vi "only_ang.vi"(9 "wanted angle":dbl=-36.7) -> ()   [LabVIEW 2019]
uses:
  <vilib>/Platform/TimedLoop/XDataNode/timing_clust.ctl
  <vilib>/Platform/TimedLoop/XDataNode/nitl_modes.ctl
  <vilib>/Platform/TimedLoop/XDataNode/wakeup.ctl
  <vilib>/FPGAPlugInAG/myRIO-1900/niLvFpga_Open_myRIO-1900.vi
  <vilib>/rvi/interface/common/dynamic/niFpgaDynamicAddResources.vi
  <vilib>/Utility/error.llb/Error Cluster From Error Code.vi
  <vilib>/rvi/errors/niLvFpgaAdjustHostInterfaceError.vi
  <vilib>/FPGAPlugInAG/Dynamic/niLvFpga_Close_Dynamic.vi
  <vilib>/rvi/interface/nirviOpenFPGA/nirviOpenFPGA.xnode
  FPGA Bitfiles/capstone_FPGATarget_FPGA(test)_jvt0Tj5QNIc.lvbitx
  FPGA(test)_.vi
  <vilib>/rvi/interface/nirviReadWriteControl/nirviReadWriteControl.xnode
  <vilib>/Platform/TimedLoop/XDataNode/XDataNode.xnode
  <vilib>/rvi/interface/nirviCloseFPGA/nirviCloseFPGA.xnode
  <vilib>/Platform/TimedLoop/XDataNode/XDNodeRunTimeDep.lvlib
  <vilib>/rvi/interface/Simulation/niFpgaSimulationCallBeginRW.vi
  NiFpgaLv.dll
panel:
  out "reference":cluster{"wanted angle":dbl, dbl}(graph)={"wanted angle"=-36.7, -36.61462118459303}
  in  "Ki":dbl=50.0
  out "pwm_out":i32
  in  "Kd":dbl=0.01
  out "방향":bool
  in  "stop":bool
  in  "Enable (escon)":bool
  out "u(k) = pwm":dbl
  in  "Kp":dbl=500.0
  out "now angle":dbl
  out "Now mot rev":dbl
  out "Timeout":i32=-1
  out "Encoder  (4x)":i32
  # "쓰지마"
  # "----마이너스------해야함"
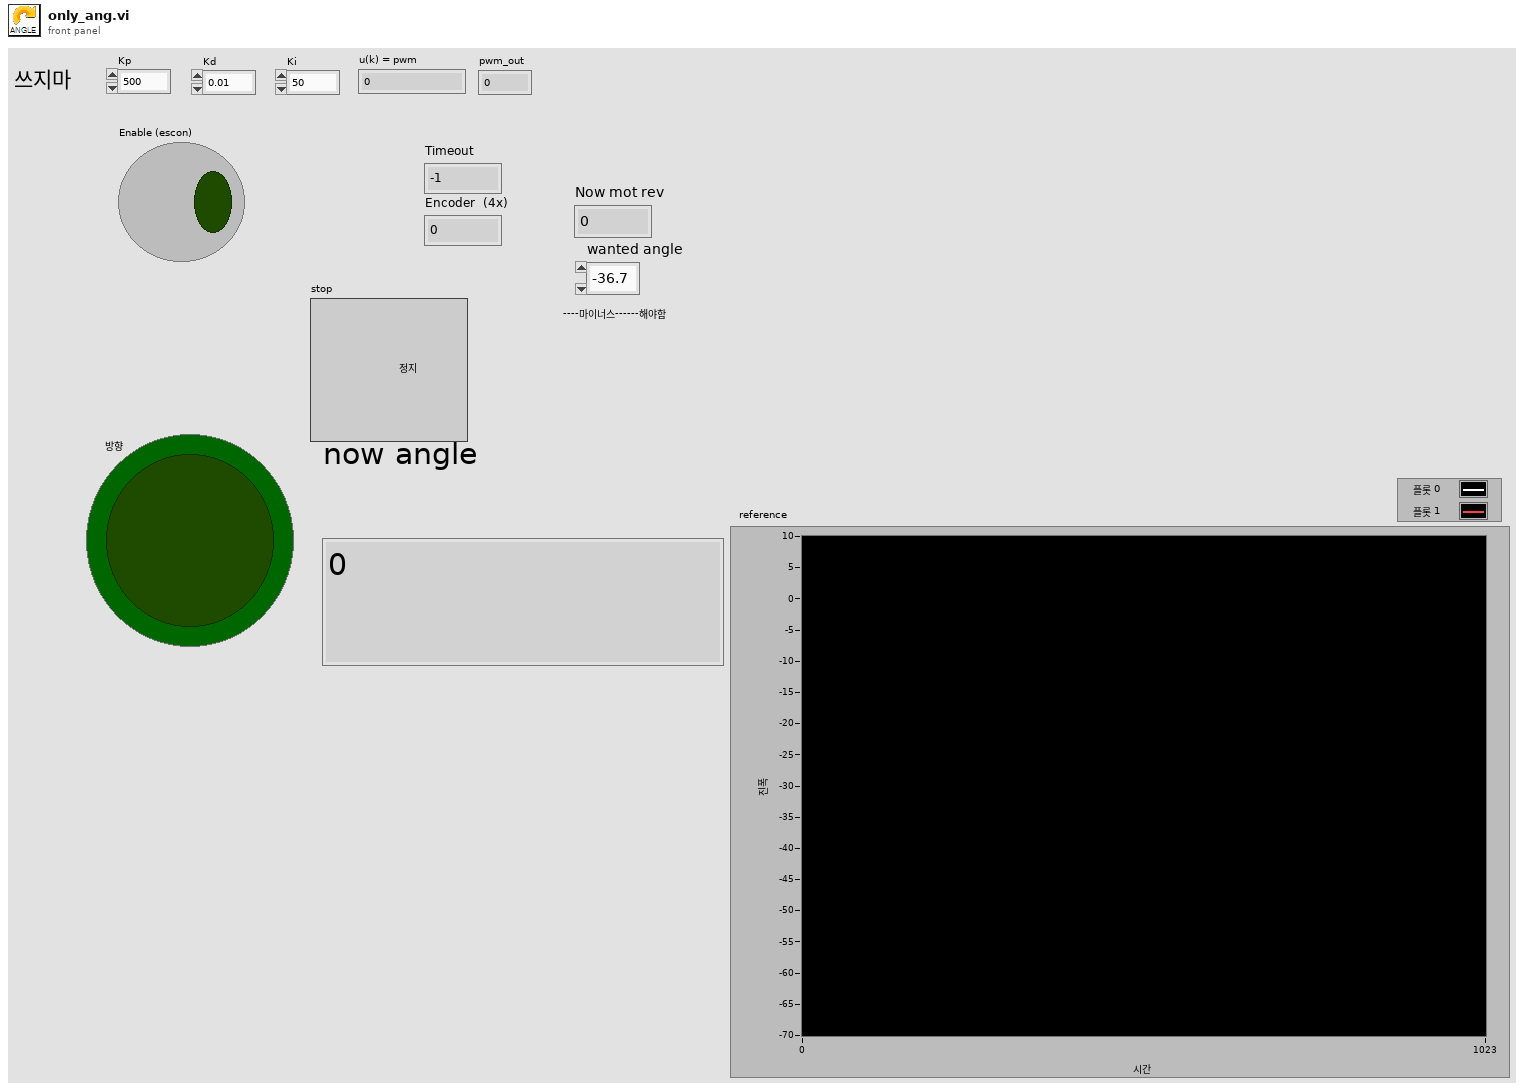
[diagram p1: front panel]
types:
  T1 = typedef "XDNodeRunTimeDep.lvlib/timing_clust.ctl" = cluster{"Expected End [f-1]":u64, "Actual End [f-1]":u64, "Finished Late? [f-1]":bool, "Expected End [i-1]":u64, "Actual End [i-1]":u64, "Finished Late? [i-1]":bool, "Expected Start [i]":u64, "Actual Start [i]":u64, "Expected Start [f]":u64, "Actual Start [f]":u64, "Source Name":string, "Structure Name":string, "Period":i64, "Deadline":i64, "Offset":i64, "Start":i64, "Priority":i32, "Timeout":i32, "Mode":T2, "Wakeup Reason":T3, "Error":errorcluster, "Source Type":string, "Secondary Source Type":string, "Global End Time":u64, "Global Start Time":u64, "Frame Duration":u64, "Iteration Duration":u64, "Assigned CPU":i32, "I/O Scan Engine Mode":u32}
  T2 = typedef "XDNodeRunTimeDep.lvlib/nitl_modes.ctl" = enum32{"No Change", "Process missed periods, maintain original phase", "Discard missed periods, maintain original phase", "Process missed periods, ignore original phase", "Discard missed periods, ignore original phase"}
  T3 = typedef "XDNodeRunTimeDep.lvlib/wakeup.ctl" = enum32{"Normal", "Aborted", "Asynchronous wakeup", "Timing source error", "Timed loop error", "Timeout"}
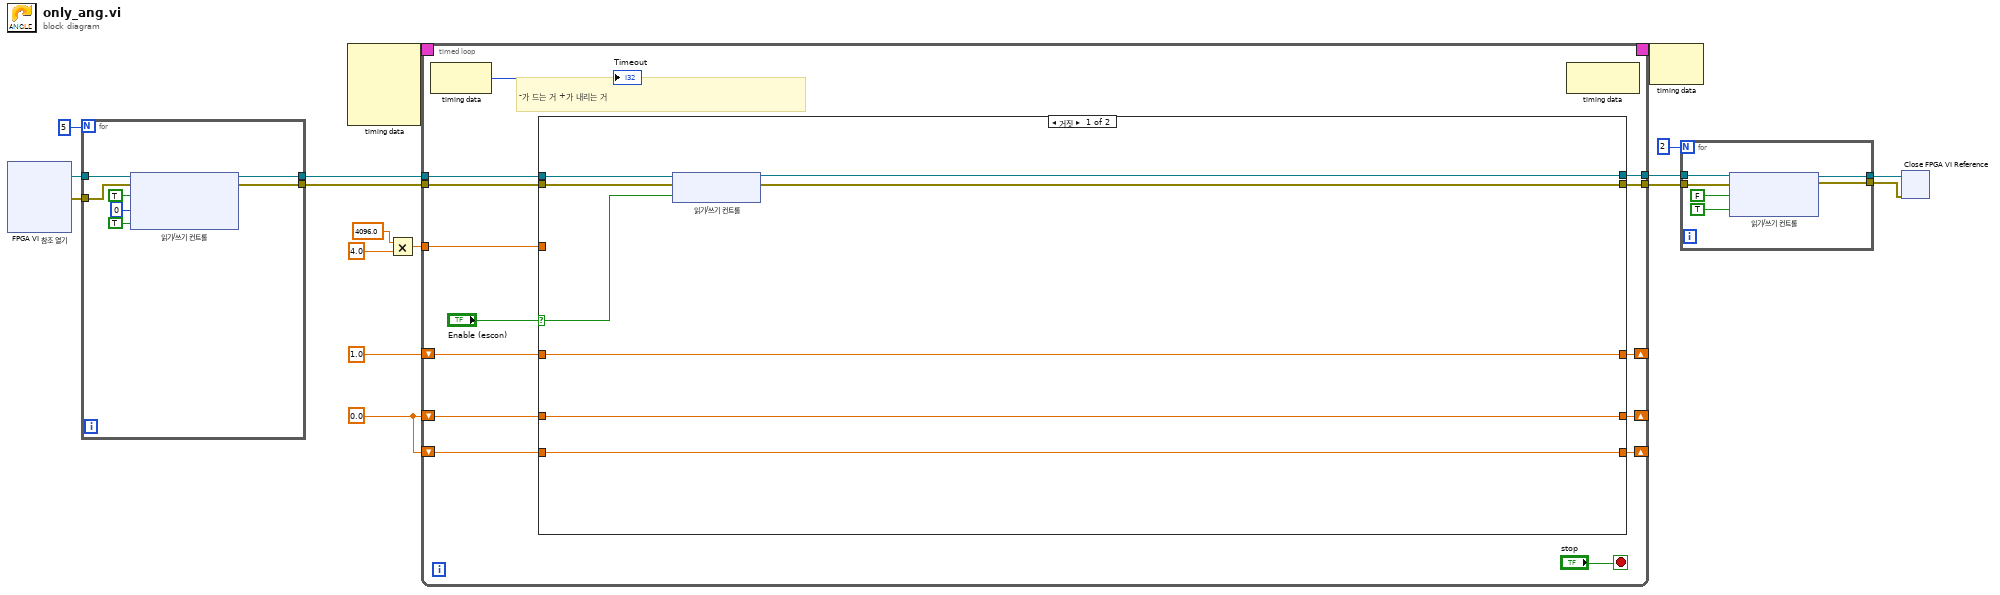
[diagram p0: block diagram]
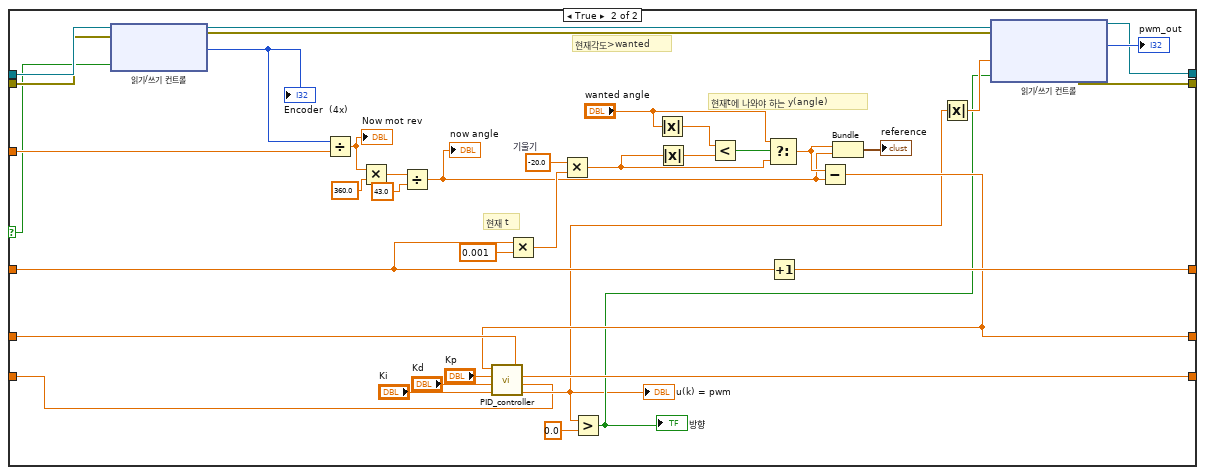
[diagram p2: hidden frame]
diagram:
  w2 = 0.0
  n1 = xnode "FPGA VI 참조 열기"() -> ("FPGA VI 참조 출력"=w14:refnum<k20>, "에러 출력"=w13:errorcluster)  [unwired: 2 in]
  n2 = for {
    N: 5 -> [_]
    tunnel: [w24] -> w10
    tunnel: [w23] -> w9
    tunnel: w14 -> [w22]
    tunnel: w13 -> [w21]
    n3 = xnode "읽기/쓰기 컨트롤"("FPGA VI 참조 입력"=w22, "에러 입력"=w21, "Enable (escon)"=TRUE, "pwm input(escon)"=0, "encoder reset"=TRUE) -> ("FPGA VI 참조 출력"=w24:refnum<k20>, "에러 출력"=w23:errorcluster)
  }
  n4 = node-c288() -> (w8:T1)  [unwired: 4 in]
  n5 = Multiply(x=4096.0, y=4.0) -> (x*y=w4:dbl)
  n6 = timed-loop {
    timing: w8 -> [_]
    timing-out: [_] -> w7
    tunnel: [w34] -> w16
    tunnel: w4 -> [w37]
    shift-right: [w36] -> _
    shift-left: w2 -> [w29]
    shift-right: [w30] -> _
    shift-left: w2 -> [w35]
    shift-right: [w32] -> _
    shift-left: 1.0 -> [w31]
    tunnel: w10 -> [w28]
    tunnel: w9 -> [w27]
    tunnel: [w25] -> w1
    stop <- "stop" stop-if-true
    # "-가 드는 거 +가 내리는 거"
    n7 = node-c288() -> (→"Timeout":i32)  [unwired: 1 in]
    n8 = case shown="거짓" "Enable (escon)" {
      selector: "Enable (escon)" -> [w39 w51]
      tunnel: w37 -> [_ w81]
      tunnel: [w44 w79] -> w36
      tunnel: w35 -> [w45 w78]
      tunnel: [w40 w75] -> w34
      tunnel: [w46 w69] -> w32
      tunnel: w31 -> [w46 w68]
      tunnel: [w45 w64] -> w30
      tunnel: w29 -> [w44 w59]
      tunnel: w28 -> [w43 w53]
      tunnel: w27 -> [w42 w52]
      tunnel: [w41 w50] -> w25
      frame False {
        n9 = xnode "읽기/쓰기 컨트롤"("FPGA VI 참조 입력"=w43, "에러 입력"=w42, "Enable (escon)"=w39) -> ("FPGA VI 참조 출력"=w41:refnum<k20>, "에러 출력"=w40:errorcluster)
      }
      frame True {
        w70 = -20.0  # 기울기
        # "현재각도>wanted"
        # "현재t에 나와야 하는 y(angle)"
        # "현재 t"
        n10 = xnode "읽기/쓰기 컨트롤"("FPGA VI 참조 입력"=w53, "에러 입력"=w52, "Enable (escon)"=w51) -> ("FPGA VI 참조 출력"=w74:refnum<k20>, "에러 출력"=w73:errorcluster, "Encoder  (4x)"=w71:i32)
        "Encoder  (4x)" <- w71
        n11 = Divide(x=w71, y=w81) -> (x/y=w82:dbl)
        "Now mot rev" <- w82
        n12 = Multiply(x=w82, y=360.0) -> (x*y=w54:dbl)
        n13 = Divide(x=w54, y=43.0) -> (x/y=w48:dbl)
        "now angle" <- w48
        n14 = Multiply(x=w68, y=0.001) -> (x*y=w66:dbl)
        n15 = Multiply(x=w70, y=w66) -> (x*y=w57:dbl)
        n16 = Absolute Value(x="wanted angle") -> (abs(x)=w56:dbl)
        n17 = Absolute Value(x=w57) -> (abs(x)=w55:dbl)
        n18 = Less?(x=w56, y=w55) -> (x < y?=w65:bool)
        n19 = Select(t="wanted angle", s=w65, f=w57) -> (s? t:f=w49:dbl)
        n20 = Increment(x=w68) -> (x+1=w69:dbl)
        n21 = Subtract(x=w49, y=w48) -> (x-y=w64:dbl)
        n22 = call "PID_controller.vi"("Error_Sum(k-1)"=w59, "Error(k-1)"=w78, "Ki"="Ki", "Kd"="Kd", "Kp"="Kp", "Error(k)"=w64) -> ("u(k)"=w61:dbl, "Error_Sum(k)"=w79:dbl)
        "u(k) = pwm" <- w61
        n23 = Greater?(x=w61, y=0.0) -> (0:w62:bool)
        "방향" <- w62
        n24 = Bundle("wanted angle"=w49, w48) -> (→"reference":cluster{"wanted angle":dbl, dbl})  [unwired: 1 in]
        n25 = Absolute Value(x=w61) -> (abs(x)=w63:dbl)
        n26 = xnode "읽기/쓰기 컨트롤"("FPGA VI 참조 입력"=w74, "에러 입력"=w73, "pwm input(escon)"=w63, "angle_DIR"=w62) -> ("FPGA VI 참조 출력"=w50:refnum<k20>, "에러 출력"=w75:errorcluster, "pwm_out"=→"pwm_out":i32)
      }
    }
    n27 = node-c288() -> ()  [unwired: 1 in, 1 out]
  }
  n28 = node-c288(w7) -> ()  [unwired: 1 out]
  n29 = for {
    N: 2 -> [_]
    tunnel: w16 -> [w93]
    tunnel: [w92] -> w12
    tunnel: [w91] -> w11
    tunnel: w1 -> [w88]
    n30 = xnode "읽기/쓰기 컨트롤"("FPGA VI 참조 입력"=w88, "에러 입력"=w93, "Enable (escon)"=FALSE, "encoder reset"=TRUE) -> ("FPGA VI 참조 출력"=w92:refnum<k20>, "에러 출력"=w91:errorcluster)
  }
  n31 = xnode "Close FPGA VI Reference"("FPGA VI 참조 입력"=w12, "에러 입력"=w11) -> ()  [unwired: 1 out]
